vi "Create.vi"(8 "error in (no error)":errorcluster, 11 "Identifier (ID, IP etc)":string) -> (0 "error out":errorcluster, 3 "Camera out":refnum<class "Camera.lvclass">)   [LabVIEW 2020, in "device.lvlib" / "Camera.lvclass"]
uses:
  Camera.lvclass
  Camera.lvclass/Camera.ctl
  bin/gindustrialcam_32-1.dll
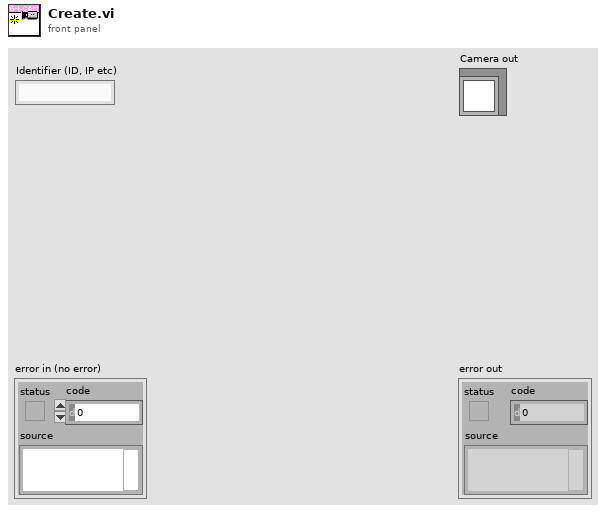
[diagram p1: front panel]
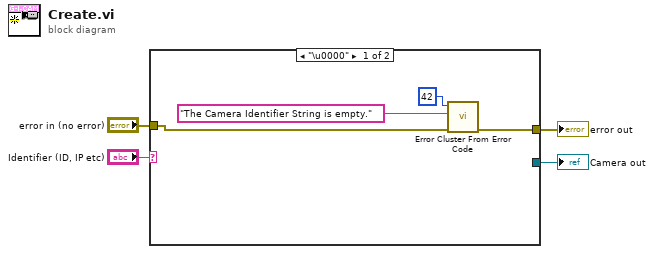
[diagram p0: block diagram]
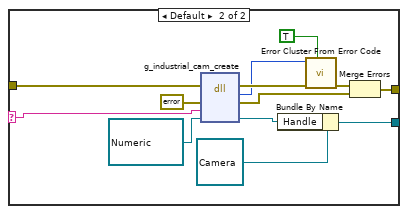
[diagram p2: hidden frame]
diagram:
  n1 = case shown="\"\"" "Identifier (ID, IP etc)" {
    selector: "Identifier (ID, IP etc)" -> [_ w12]
    tunnel: "error in (no error)" -> [w8 w21]
    tunnel: [w7 w14] -> w3
    tunnel: [_ w10] -> w1
    frame "\u0000" {
      n2 = call <vilib>:"Error Cluster From Error Code.vi"("error in (no error)"=w8, "error message (\"\")"="The Camera Identifier String is empty." ("error message (\"\")"), "error code (0)"=42) -> ("error out"=w7:errorcluster)  [unwired: 6 in]
    }
    frame Default {
      n3 = dll-call lib="C:/Workspace/SSDC/g-industrial-camera/LabVIEW/bin/gindustrialcam_32-1.dll" fn="g_industrial_cam_create"(error in=w21, "err"=errorcluster {"status"=FALSE, "code"=0, "source"=""} ("error constant"), "Identifier"=w12, "edvr"=refnum<data-value> refnum ("data value reference")) -> (error out=w20:errorcluster, "Mg_Error"=w19:i32, "err"=w17:errorcluster, "edvr"=w11:refnum<data-value>)  [unwired: 3 in, 1 out]
      n4 = Bundle By Name(cluster=refnum<class "Camera.lvclass"> refnum ("Camera out"), "Handle"=w11) -> (w10:refnum<class "Camera.lvclass">)
      n5 = call <vilib>:"Error Cluster From Error Code.vi"("show call chain? (False)"=TRUE, "error in (no error)"=w20, "error code (0)"=w19) -> ("error out"=w18:errorcluster)  [unwired: 6 in]
      n6 = Merge Errors(w18, w17) -> (w14:errorcluster)
    }
  }
  "error out" <- w3
  "Camera out" <- w1
